vi "Zero Phase Filtering.vi"() -> ()   [LabVIEW 2020]
doc: "Demonstrates the difference between filters implemented using the FIR Filter VI and the Zero Phase Filter VI."
uses:
  <vilib>/Analysis/3filter.llb/Zero Phase Filter (DBL).vi
  <vilib>/Analysis/3filter.llb/FIR Filter (DBL).vi
  <vilib>/Analysis/NI_AALBase.lvlib
panel:
  out "Results":dbl[][](graph)
  # "Overview: Demonstrates the difference between filters implemented using the FIR Filter VI and the Zero Phase Filter VI.\nRequirements: LabVIEW Full Development System\nInstructions: \n1. Run the VI.\n2. Observe the original noisy signal, the FIR Filter results, and the Zero Phase Filter results in the Results graph."
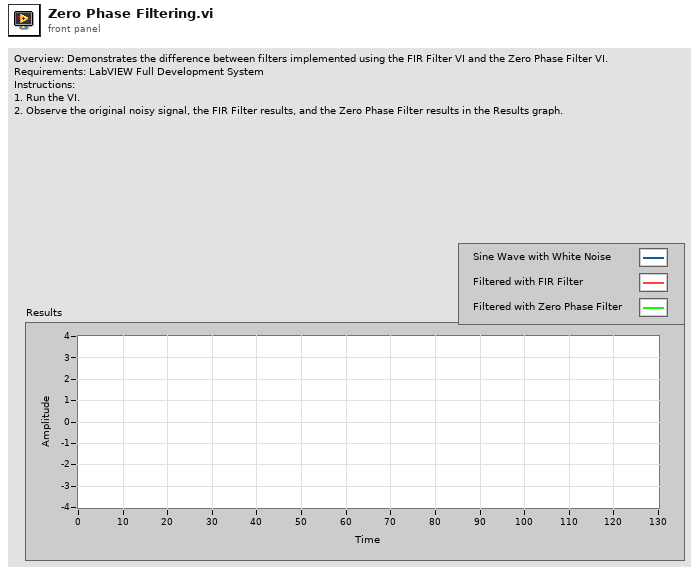
[diagram p1: front panel]
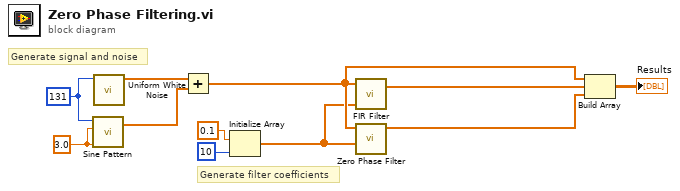
[diagram p0: block diagram]
diagram:
  w1 = 3.0
  w11 = 131 ("samples")
  # "Generate filter coefficients"
  # "Generate signal and noise"
  n1 = call <vilib>:"Sine Pattern.vi"("cycles"=w1, "amplitude"=w1, "samples"=w11) -> ("Sinusoidal Pattern"=w9:dbl[])  [unwired: 1 in, 1 out]
  n2 = call <vilib>:"Uniform White Noise.vi"("samples"=w11) -> ("uniform white noise"=w10:dbl[])  [unwired: 9 in, 1 out]
  n3 = Add(x=w10, y=w9) -> (x+y=w5:dbl[])
  n4 = Initialize Array(0.1 ("element"), 10 ("dimension size")) -> (w4:dbl[])
  n5 = call-poly <vilib>:"FIR Filter.vi"("FIR Coefficients"=w4, "X"=w5) -> ("Filtered X"=w3:dbl[])  [unwired: 2 in, 1 out]
  n6 = call-poly <vilib>:"Zero Phase Filter.vi"("Forward Coefficients"=w4, "X"=w5) -> ("Filtered X"=w2:dbl[])  [unwired: 8 in, 1 out]
  n7 = Build Array(w5, w3, w2) -> (→"Results":dbl[][])
